vi "StoreInFileString.vi"(0 "element0":string="data", 1 "element 5":string, 2 "element 6":string, 3 "element 7":string, 4 "element 8":string, 5 "element1":string, 6 "element 9":string, 7 "element 2":string, 8 "element 10":string, 9 "element 3":string, 10 "element 11":string, 11 "element 4":string, 12 "FileName":string="data", 13 "element 14":string, 14 "element 13":string, 15 "element 12":string) -> ()   [LabVIEW 2018]
uses:
  <vilib>/Utility/file.llb/Write Delimited Spreadsheet (string).vi
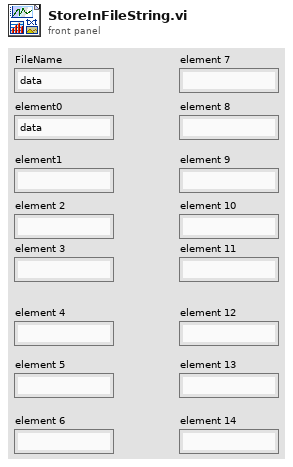
[diagram p1: front panel]
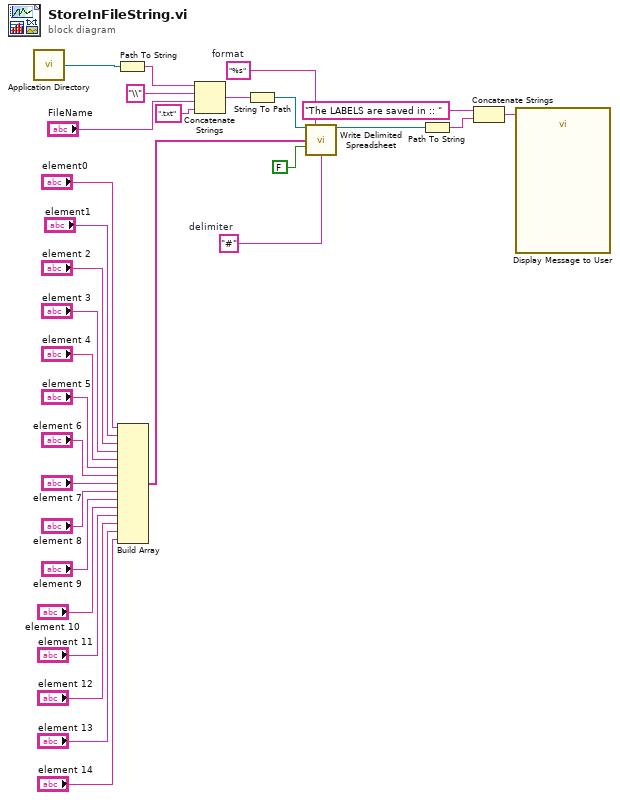
[diagram p0: block diagram]
diagram:
  w24 = "%s"  # format
  w23 = "#"  # delimiter
  n1 = call <vilib>:"Application Directory.vi"() -> ("Application Directory"=w22:path)
  n2 = Path To String(path=w22) -> (string=w26:string)
  n3 = Build Array("element0", "element1", "element 2", "element 3", "element 4", "element 5", "element 6", "element 7", "element 8", "element 9", "element 10", "element 11", "element 12", "element 13", "element 14") -> (w1:string[])
  n4 = Concatenate Strings(w26, "\\" ("string"), "FileName", ".txt" ("string")) -> (w29:string)
  n5 = String To Path(string=w29) -> (path=w27:path)
  n6 = call-poly <vilib>:"Write Delimited Spreadsheet.vi"("file path (dialog if empty)"=w27, "format (%s)"=w24, "1D data"=w1, "append to file? (new file:F)"=FALSE, "delimiter (\\t)"=w23) -> ("new file path (Not A Path if cancelled)"=w25:path)  [unwired: 9 in, 1 out]
  n7 = Path To String(path=w25) -> (string=w18:string)
  n8 = Concatenate Strings("The LABELS are saved in :: " ("string"), w18) -> (w19:string)
  n9 = call "Display Message to User"("Message"=w19) -> ()  [unwired: 9 in, 2 out]
